vi "hcam_environment_monitor.vi"() -> ()   [LabVIEW 2020]
uses:
  <vilib>/Instr/_visa.llb/VISA Configure Serial Port (Instr).vi
panel:
  out "Connected":bool
  out "Response":string
  in  "CONNECTION":bool
  out "Bytes Read":u32
  in  "VISA Resource":refnum<visa-resource-name>="COM1"
  in  "Tab Control":enum32{"Page 1", "Page 2"}(tab)
  in  "End":timestamp caption="Day End" format="%<%H:%M>T"
  in  "Start":timestamp caption="Day Start" format="%<%H:%M>T"
  in  "SEND LED":bool caption="Boolean"
  out "Color Box":u32(colorbox)
  in  "R":u8
  in  "G":u8
  in  "B":u8
  in  "SEND RTC":bool caption="Boolean"
  in  "SEND INT":bool caption="Boolean"
  in  "INT 2":u8 caption="Brightness"
  out "Humidity":string caption="Humidity (%)"
  out "Temp":string caption="Temp (°C)"
  out "Temp 2":string caption="Temp (°C)"
  in  "B 2":u8 caption="B"
  in  "G 2":u8 caption="G"
  in  "R 2":u8 caption="R"
  out "Color Box 2":u32(colorbox)
  in  "SEND RTC 2":bool caption="Boolean"
  in  "SEND LED 2":bool caption="Boolean"
  in  "End 2":timestamp caption="Day End" format="%<%H:%M>T"
  in  "Start 2":timestamp caption="Day Start" format="%<%H:%M>T"
  in  "SEND INT 2":bool caption="Boolean"
  in  "INT":u8 caption="Brightness"
  out "Humidity 2":string caption="Humidity (%)"
  # "Serial Monitor"
  # "--- Box 1 ---"
  # "Auto LED Timer"
  # "Manual Color Control"
  # "Climate Readings"
  # "--- Box 2 ---"
  # "Auto LED Timer"
  # "Manual Color Control"
  # "Climate Readings"
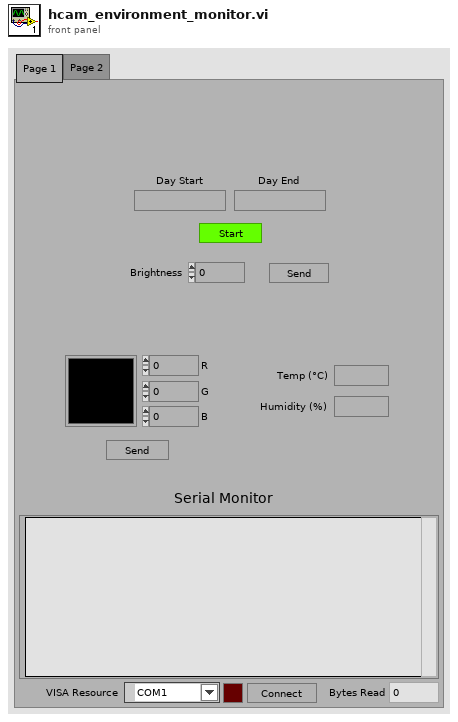
[diagram p1: front panel]
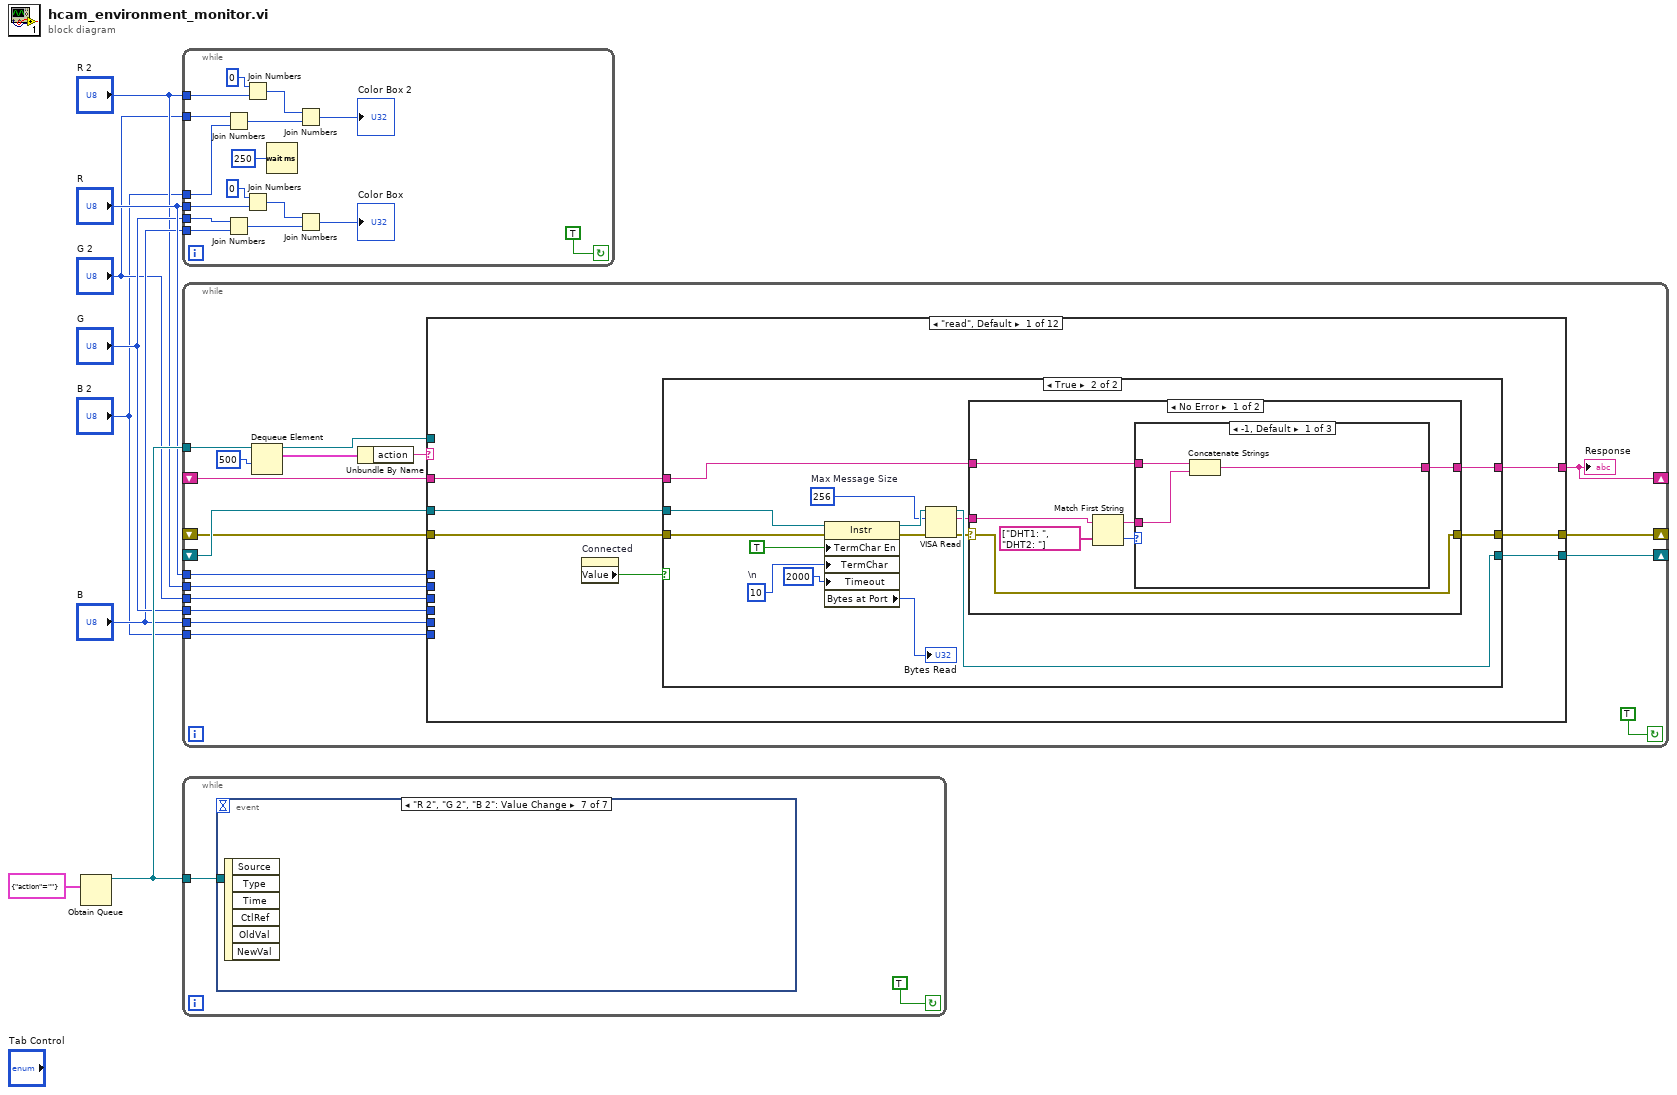
[diagram p0: block diagram]
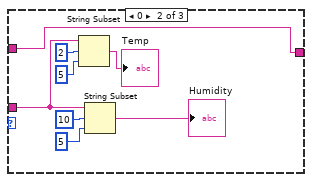
[diagram p3: hidden frame]
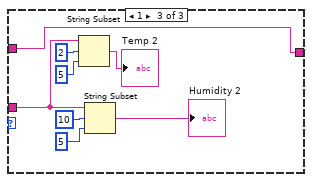
[diagram p4: hidden frame]
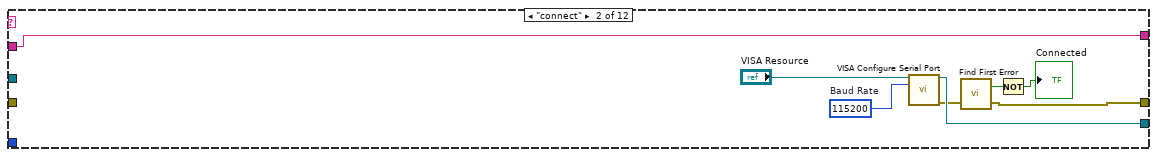
[diagram p6: hidden frame]
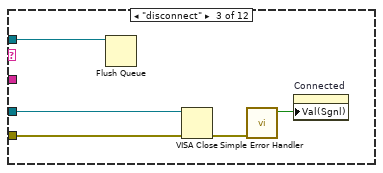
[diagram p7: hidden frame]
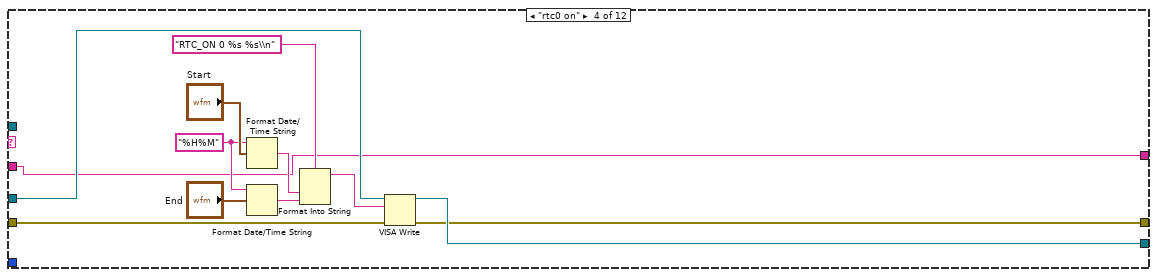
[diagram p8: hidden frame]
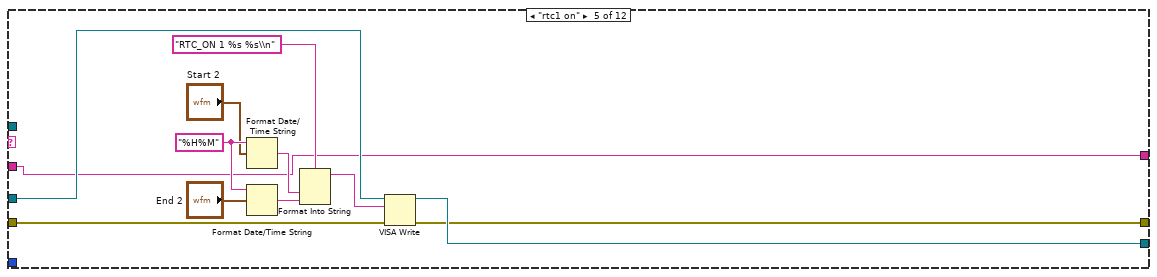
[diagram p9: hidden frame]
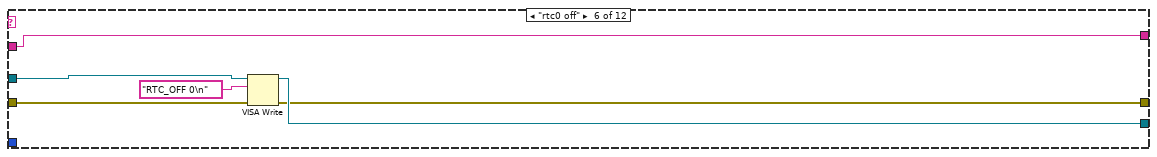
[diagram p10: hidden frame]
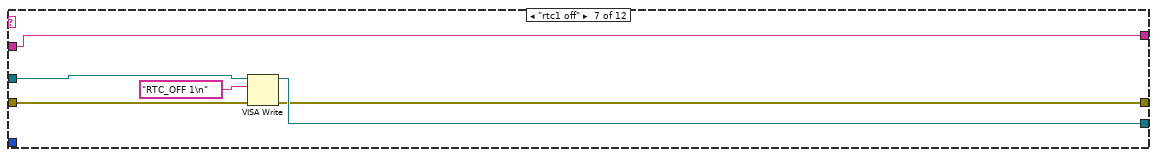
[diagram p11: hidden frame]
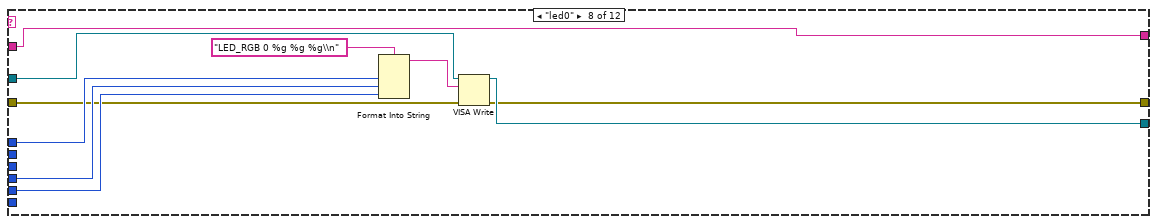
[diagram p12: hidden frame]
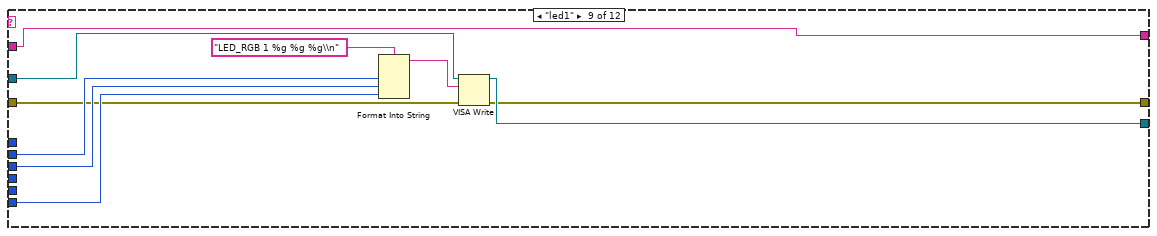
[diagram p13: hidden frame]
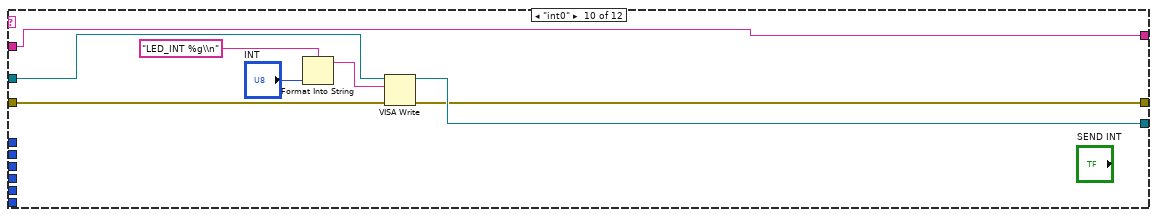
[diagram p14: hidden frame]
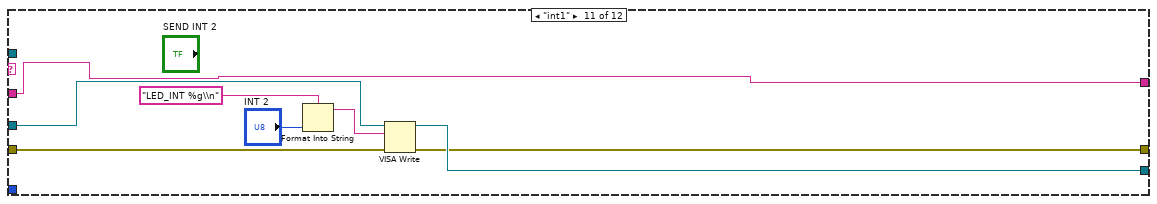
[diagram p15: hidden frame]
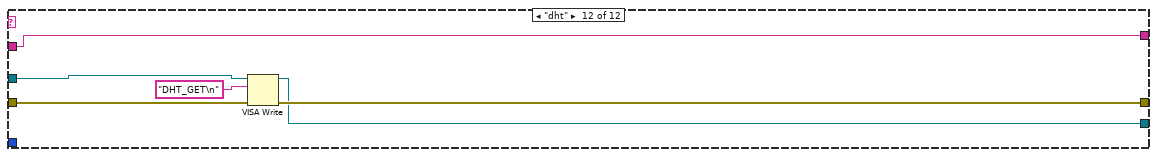
[diagram p16: hidden frame]
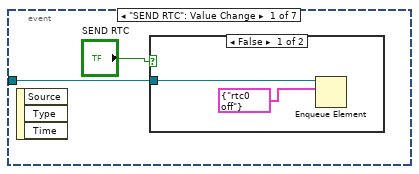
[diagram p17: hidden frame]
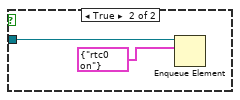
[diagram p18: hidden frame]
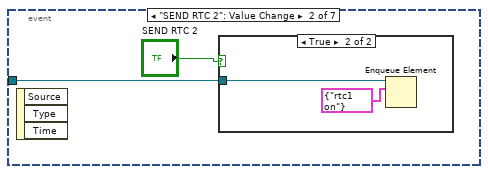
[diagram p19: hidden frame]
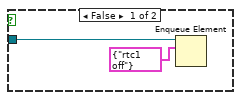
[diagram p20: hidden frame]
diagram:
  n1 = Obtain Queue(element data type=cluster{"action":string} {"action"=""}) -> (queue out=w7:refnum<queue>)  [unwired: 4 in, 2 out]
  n2 = while {
    tunnel: "R" -> [w18]
    tunnel: "G" -> [w17]
    tunnel: "B" -> [w16]
    tunnel: "R 2" -> [w14]
    tunnel: "G 2" -> [w12]
    tunnel: "B 2" -> [w11]
    stop <- TRUE continue-if-true
    n3 = Join Numbers(hi=w12, lo=w11) -> ((hi.lo)=w10:u16)
    n4 = Join Numbers(hi=w17, lo=w16) -> ((hi.lo)=w20:u16)
    n5 = Join Numbers(hi=u8 0, lo=w14) -> ((hi.lo)=w9:u16)
    n6 = Join Numbers(hi=u8 0, lo=w18) -> ((hi.lo)=w21:u16)
    n7 = Wait (ms)(milliseconds to wait=u32 250) -> ()  [unwired: 1 out]
    n8 = Join Numbers(hi=w9, lo=w10) -> ((hi.lo)=→"Color Box 2":u32)
    n9 = Join Numbers(hi=w21, lo=w20) -> ((hi.lo)=→"Color Box":u32)
  }
  n10 = while {
    tunnel: w7 -> [w42]
    shift-right: [w37] -> _
    shift-left: _ -> [w36]
    shift-right: [w35] -> _
    shift-left: _ -> [w34]
    tunnel: "R" -> [w33]
    tunnel: "G" -> [w32]
    tunnel: "B" -> [w31]
    tunnel: "R 2" -> [w30]
    tunnel: "G 2" -> [w29]
    tunnel: "B 2" -> [w28]
    shift-right: [w26] -> _
    shift-left: _ -> [w27]
    stop <- TRUE continue-if-true
    n11 = Dequeue Element(queue=w42, timeout in ms (-1)=500) -> (queue out=w38:refnum<queue>, element=w40:cluster{"action":string})  [unwired: 1 in, 2 out]
    n12 = Unbundle By Name(w40) -> ("action"=w39:string)
    n13 = case shown="\"read\", Default" w39 {
      tunnel: w38 -> [_ _ w101 _ _ _ _ _ _ _ _ _]
      tunnel: [w43 w97 _ w108 w121 w133 w139 w147 w157 w164 w173 w178] -> w37
      tunnel: w36 -> [w49 _ w104 w109 w120 w134 w140 w148 w158 w165 w174 w179]
      tunnel: [w47 w95 _ w106 w118 w131 w137 w142 w152 w162 w170 w180] -> w35
      tunnel: w34 -> [w48 _ w102 w107 w119 w132 w138 w143 w153 w163 w171 w181]
      tunnel: w33 -> [_ _ _ _ _ _ _ w146 _ _ _ _]
      tunnel: w32 -> [_ _ _ _ _ _ _ w145 _ _ _ _]
      tunnel: w31 -> [_ _ _ _ _ _ _ w144 _ _ _ _]
      tunnel: w30 -> [_ _ _ _ _ _ _ _ w156 _ _ _]
      tunnel: w29 -> [_ _ _ _ _ _ _ _ w155 _ _ _]
      tunnel: w28 -> [_ _ _ _ _ _ _ _ w154 _ _ _]
      tunnel: [w45 w92 _ w105 w117 w130 w136 w141 w151 w161 w169 w182] -> w26
      tunnel: w27 -> [w46 w92 _ w105 w117 w130 w136 w141 w151 w161 w169 w182]
      frame "read", Default {
        n14 = property on="Connected" class="Bool (strict)"() -> ("Value"=w44:bool)  [unwired: 2 in, 2 out]
        n15 = case shown="True" w44 {
          tunnel: w49 -> [_ w57]
          tunnel: w48 -> [_ w56]
          tunnel: [_ w50] -> w47
          tunnel: w46 -> [_ w53]
          tunnel: [_ w51] -> w45
          tunnel: [_ w55] -> w43
          frame False {
          }
          frame True {
            w61 = u32 256  # Max Message Size
            w59 = u8 10  # \n
            n16 = property class="Instr"(reference=w57, error in=w56, "TermChar En"=TRUE ("Message Based Settings:Termination Character Enable"), "TermChar"=w59, "Timeout"=u32 2000 ("General Settings:Timeout Value")) -> (reference out=w64:refnum<visa-resource-name>, error out=w63:errorcluster, "Bytes at Port"=→"Bytes Read":u32)
            n17 = VISA Read(VISA resource name=w64, byte count=w61, error in (no error)=w63) -> (VISA resource name out=w55:refnum<visa-resource-name>, read buffer=w52:string, error out=w54:errorcluster)  [unwired: 1 out]
            n18 = case shown="No Error" w54 {
              selector: w54 -> [w65 _]
              tunnel: w53 -> [w69 w91]
              tunnel: w52 -> [w67 _]
              tunnel: [w66 w91] -> w51
              tunnel: [w65 _] -> w50
              frame No Error {
                n19 = Match First String(2:string[] ["DHT1: ", "DHT2: "], 3:w67) -> (0:w70:i32, 1:w71:string)
                n20 = case shown="-1, Default" w70 {
                  tunnel: w71 -> [w72 w76 w85]
                  tunnel: w69 -> [w74 w82 w90]
                  tunnel: [w73 w82 w90] -> w66
                  frame -1, Default {
                    n21 = Concatenate Strings(w74, w72) -> (w73:string)
                  }
                  frame 0 {
                    n22 = String Subset(string=w76, offset (0)=2, length (rest)=5) -> (substring=→"Temp":string)
                    n23 = String Subset(string=w76, offset (0)=10, length (rest)=5) -> (substring=→"Humidity":string)
                  }
                  frame 1 {
                    n24 = String Subset(string=w85, offset (0)=2, length (rest)=5) -> (substring=→"Temp 2":string)
                    n25 = String Subset(string=w85, offset (0)=10, length (rest)=5) -> (substring=→"Humidity 2":string)
                  }
                }
              }
              frame Error {
              }
            }
          }
        }
      }
      frame "connect" {
        w98 = u32 115200  # Baud Rate
        n26 = call-poly "VISA Configure Serial Port"("VISA resource name"="VISA Resource", "baud rate (9600)"=w98) -> ("VISA resource name out"=w97:refnum<visa-resource-name>, "error out"=w96:errorcluster)  [unwired: 7 in, 5 out]
        n27 = call <vilib>:"Find First Error.vi"("error in (no error)"=w96) -> ("error out"=w95:errorcluster, "error?"=w94:bool)  [unwired: 3 in]
        n28 = Not(x=w94) -> (.not. x?=→"Connected":bool)
      }
      frame "disconnect" {
        n29 = Flush Queue(queue=w101) -> ()  [unwired: 1 in, 3 out]
        n30 = VISA Close(VISA resource name=w104, error in (no error)=w102) -> (error out=w103:errorcluster)
        n31 = call <vilib>:"Simple Error Handler.vi"("error in (no error)"=w103) -> ("error?"=w100:bool)  [unwired: 1 in, 7 out]
        n32 = property on="Connected" class="Bool (strict)"("Val(Sgnl)"=w100) -> ()  [unwired: 2 in, 2 out]
      }
      frame "rtc0 on" {
        w110 = "%H%M"
        n33 = Format Date/Time String(time format string (%c)=w110, seconds (now)="Start") -> (date/time string=w116:string)  [unwired: 1 in]
        n34 = Format Date/Time String(time format string (%c)=w110, seconds (now)="End") -> (date/time string=w115:string)  [unwired: 1 in]
        n35 = Format Into String(format string="RTC_ON 0 %s %s\\n", w116, w115) -> (resulting string=w112:string)  [unwired: 2 in, 1 out]
        n36 = VISA Write(VISA resource name=w109, write buffer=w112, error in (no error)=w107) -> (VISA resource name out=w108:refnum<visa-resource-name>, error out=w106:errorcluster)  [unwired: 1 out]
      }
      frame "rtc1 on" {
        w126 = "%H%M"
        n37 = Format Date/Time String(time format string (%c)=w126, seconds (now)="Start 2") -> (date/time string=w124:string)  [unwired: 1 in]
        n38 = Format Date/Time String(time format string (%c)=w126, seconds (now)="End 2") -> (date/time string=w125:string)  [unwired: 1 in]
        n39 = Format Into String(format string="RTC_ON 1 %s %s\\n", w124, w125) -> (resulting string=w127:string)  [unwired: 2 in, 1 out]
        n40 = VISA Write(VISA resource name=w120, write buffer=w127, error in (no error)=w119) -> (VISA resource name out=w121:refnum<visa-resource-name>, error out=w118:errorcluster)  [unwired: 1 out]
      }
      frame "rtc0 off" {
        n41 = VISA Write(VISA resource name=w134, write buffer="RTC_OFF 0\n" ("format string"), error in (no error)=w132) -> (VISA resource name out=w133:refnum<visa-resource-name>, error out=w131:errorcluster)  [unwired: 1 out]
      }
      frame "rtc1 off" {
        n42 = VISA Write(VISA resource name=w140, write buffer="RTC_OFF 1\n" ("format string"), error in (no error)=w138) -> (VISA resource name out=w139:refnum<visa-resource-name>, error out=w137:errorcluster)  [unwired: 1 out]
      }
      frame "led0" {
        n43 = Format Into String(format string="LED_RGB 0 %g %g %g\\n", w146, w145, w144) -> (resulting string=w149:string)  [unwired: 2 in, 1 out]
        n44 = VISA Write(VISA resource name=w148, write buffer=w149, error in (no error)=w143) -> (VISA resource name out=w147:refnum<visa-resource-name>, error out=w142:errorcluster)  [unwired: 1 out]
      }
      frame "led1" {
        n45 = Format Into String(format string="LED_RGB 1 %g %g %g\\n", w156, w155, w154) -> (resulting string=w159:string)  [unwired: 2 in, 1 out]
        n46 = VISA Write(VISA resource name=w158, write buffer=w159, error in (no error)=w153) -> (VISA resource name out=w157:refnum<visa-resource-name>, error out=w152:errorcluster)  [unwired: 1 out]
      }
      frame "int0" {
        n47 = Format Into String(format string="LED_INT %g\\n", "INT") -> (resulting string=w166:string)  [unwired: 2 in, 1 out]
        n48 = VISA Write(VISA resource name=w165, write buffer=w166, error in (no error)=w163) -> (VISA resource name out=w164:refnum<visa-resource-name>, error out=w162:errorcluster)  [unwired: 1 out]
      }
      frame "int1" {
        n49 = Format Into String(format string="LED_INT %g\\n", "INT 2") -> (resulting string=w175:string)  [unwired: 2 in, 1 out]
        n50 = VISA Write(VISA resource name=w174, write buffer=w175, error in (no error)=w171) -> (VISA resource name out=w173:refnum<visa-resource-name>, error out=w170:errorcluster)  [unwired: 1 out]
      }
      frame "dht" {
        n51 = VISA Write(VISA resource name=w179, write buffer="DHT_GET\n" ("format string"), error in (no error)=w181) -> (VISA resource name out=w178:refnum<visa-resource-name>, error out=w180:errorcluster)  [unwired: 1 out]
      }
    }
    "Response" <- w26
  }
  n52 = while {
    tunnel: w7 -> [w184]
    stop <- TRUE continue-if-true
    n53 = event shown="[6] \"R 2\", \"G 2\", \"B 2\": Value Change" {
      selector: _ -> [_ _ _ _ _ _ _]
      dyn-events: _ -> [_ _ _ _ _ _ _]
      timeout: _ -> [_ _ _ _ _ _ _]
      tunnel: w184 -> [w185 w191 w197 w199 w202 _ _]
      event "SEND RTC": Value Change {
        n54 = event-data() -> ()  [unwired: 1 in, 3 out]
        n55 = case shown="False" "SEND RTC" {
          tunnel: w185 -> [w187 w189]
          frame False {
            n56 = Enqueue Element(queue=w187, element=cluster{"action":string} {"action"="rtc0 off"}) -> ()  [unwired: 2 in, 3 out]
          }
          frame True {
            n57 = Enqueue Element(queue=w189, element=cluster{"action":string} {"action"="rtc0 on"}) -> ()  [unwired: 2 in, 3 out]
          }
        }
      }
      event "SEND RTC 2": Value Change {
        n58 = event-data() -> ()  [unwired: 1 in, 3 out]
        n59 = case shown="True" "SEND RTC 2" {
          tunnel: w191 -> [w193 w195]
          frame False {
            n60 = Enqueue Element(queue=w193, element=cluster{"action":string} {"action"="rtc1 off"}) -> ()  [unwired: 2 in, 3 out]
          }
          frame True {
            n61 = Enqueue Element(queue=w195, element=cluster{"action":string} {"action"="rtc1 on"}) -> ()  [unwired: 2 in, 3 out]
          }
        }
      }
      event "SEND LED": Value Change {
        n62 = event-data() -> ()  [unwired: 1 in, 3 out]
        n63 = Enqueue Element(queue=w197, element=cluster{"action":string} {"action"="led0"}) -> ()  [unwired: 2 in, 3 out]
      }
      event "SEND LED 2": Value Change {
        n64 = event-data() -> ()  [unwired: 1 in, 3 out]
        n65 = Enqueue Element(queue=w199, element=cluster{"action":string} {"action"="led1"}) -> ()  [unwired: 2 in, 3 out]
      }
      event "CONNECTION": Value Change {
        n66 = event-data() -> ()  [unwired: 1 in, 5 out]
        n67 = case shown="False" "CONNECTION" {
          tunnel: w202 -> [w203 w206]
          frame False {
            n68 = Enqueue Element(queue=w203, element=cluster{"action":string} {"action"="disconnect"}) -> ()  [unwired: 2 in, 3 out]
          }
          frame True {
            n69 = Enqueue Element(queue=w206, element=cluster{"action":string} {"action"="connect"}) -> ()  [unwired: 2 in, 3 out]
          }
        }
      }
      event "Color Box 2": Value Change {
        n70 = event-data() -> ()  [unwired: 1 in, 1 out]
      }
      event "R 2", "G 2", "B 2": Value Change {
        n71 = event-data() -> ()  [unwired: 1 in, 6 out]
      }
    }
  }
